vi "Send Abstract Message.vi"(8 "error in":errorcluster, 10 "AbstractMessage":T1, 11 "Engine in":refnum<class "Engine.lvclass">) -> (0 "error out":errorcluster, 3 "Engine out":refnum<class "Engine.lvclass">)   [LabVIEW 2023, in "Engine.lvlib" / "Engine.lvclass"]
uses:
  Library/Engine.lvclass
  Custom Controls/AbstractMessage.ctl
  Library/Engine.lvclass/Engine.ctl
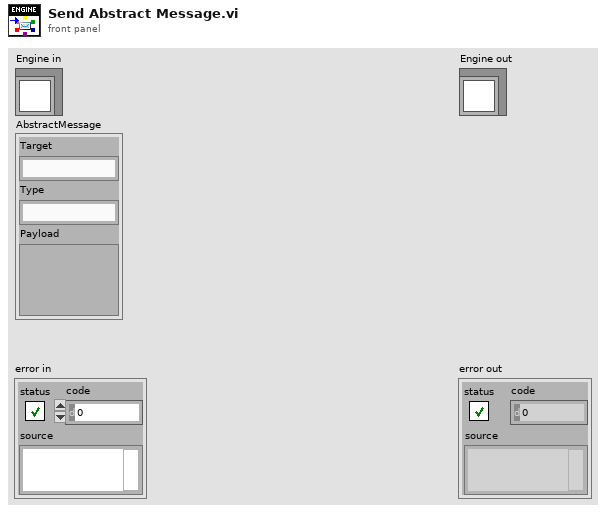
[diagram p1: front panel]
types:
  T1 = typedef "Engine.lvlib/Engine.lvclass/AbstractMessage.ctl" = cluster{"Target":string, "Type":string, "Payload":variant}
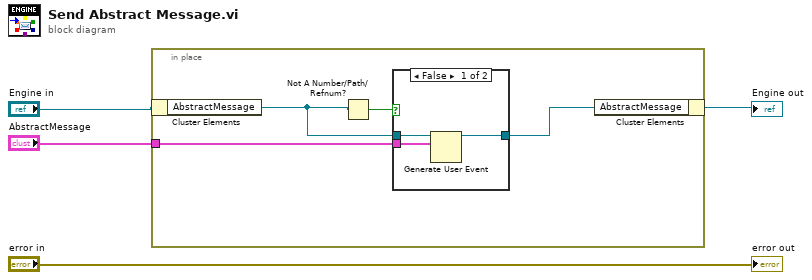
[diagram p0: block diagram]
diagram:
  n1 = in-place {
    in-place-border: "AbstractMessage" -> [w7]
    n2 = in-place-cluster #1("Engine in") -> ("AbstractMessage"=w6:refnum<user-event>)
    n3 = Not A Number/Path/Refnum?(number/path/refnum=w6) -> (NaN/Path/Refnum?=w5:bool)
    n4 = case shown="False" w5 {
      tunnel: [w11 w12] -> w8
      tunnel: w7 -> [w10 _]
      tunnel: w6 -> [w9 w12]
      frame False {
        n5 = Generate User Event(user event=w9, event data cluster=w10) -> (user event out=w11:refnum<user-event>)  [unwired: 2 in, 1 out]
      }
      frame True {
      }
    }
    n6 = in-place-cluster #1("AbstractMessage"=w8) -> (→"Engine out":refnum<class "Engine.lvclass">)
  }
  "error out" <- "error in"
